vi "Read Joystick.vi"(8 "Joystick Deadbanded Value (default of 0.1)":dbl, 11 "Joystick L 1 DevRef":T1) -> (1 "Joystick L 2 X Axis":dbl, 2 "Joystick L 1 Y Axis":dbl, 3 "Joystick L 1 X Axis":dbl)   [LabVIEW 2014]
uses:
  <vilib>/Rock Robotics/WPI/Joystick/WPI_JoystickDevRef.ctl
  <vilib>/Rock Robotics/WPI/Joystick/WPI_JoystickDeviceEnum.ctl
  Global Variables.vi
  <vilib>/Rock Robotics/WPI/Joystick/WPI_JoystickGetSetRefNum.vi
  <vilib>/Rock Robotics/Network Tables/SD Write Number.vi
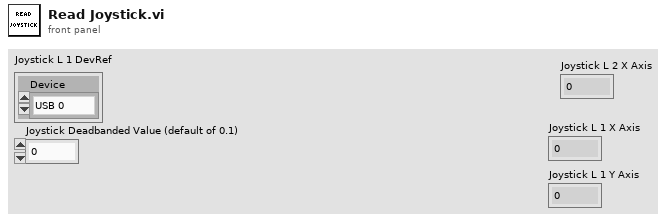
[diagram p1: front panel]
types:
  T1 = typedef "WPI_JoystickDevRef.ctl" = cluster{"Device":T2}
  T2 = typedef "WPI_JoystickDeviceEnum.ctl" = enum16{"USB 0", "USB 1", "USB 2", "USB 3", "USB 4", "USB 5"}
  T3 = cluster{"Buttons[0]":bool, "Buttons[1]":bool, "Buttons[2]":bool, "Buttons[3]":bool, "Buttons[4]":bool, "Buttons[5]":bool, "Buttons[6]":bool, "Buttons[7]":bool, "Buttons[8]":bool}
  T4 = cluster{"Axes[0]":dbl, "Axes[1]":dbl, "Axes[2]":dbl, "Axes[3]":dbl, "Axes[4]":dbl, "Axes[5]":dbl, "Axes[6]":dbl, "Axes[7]":dbl, "Axes[8]":dbl}
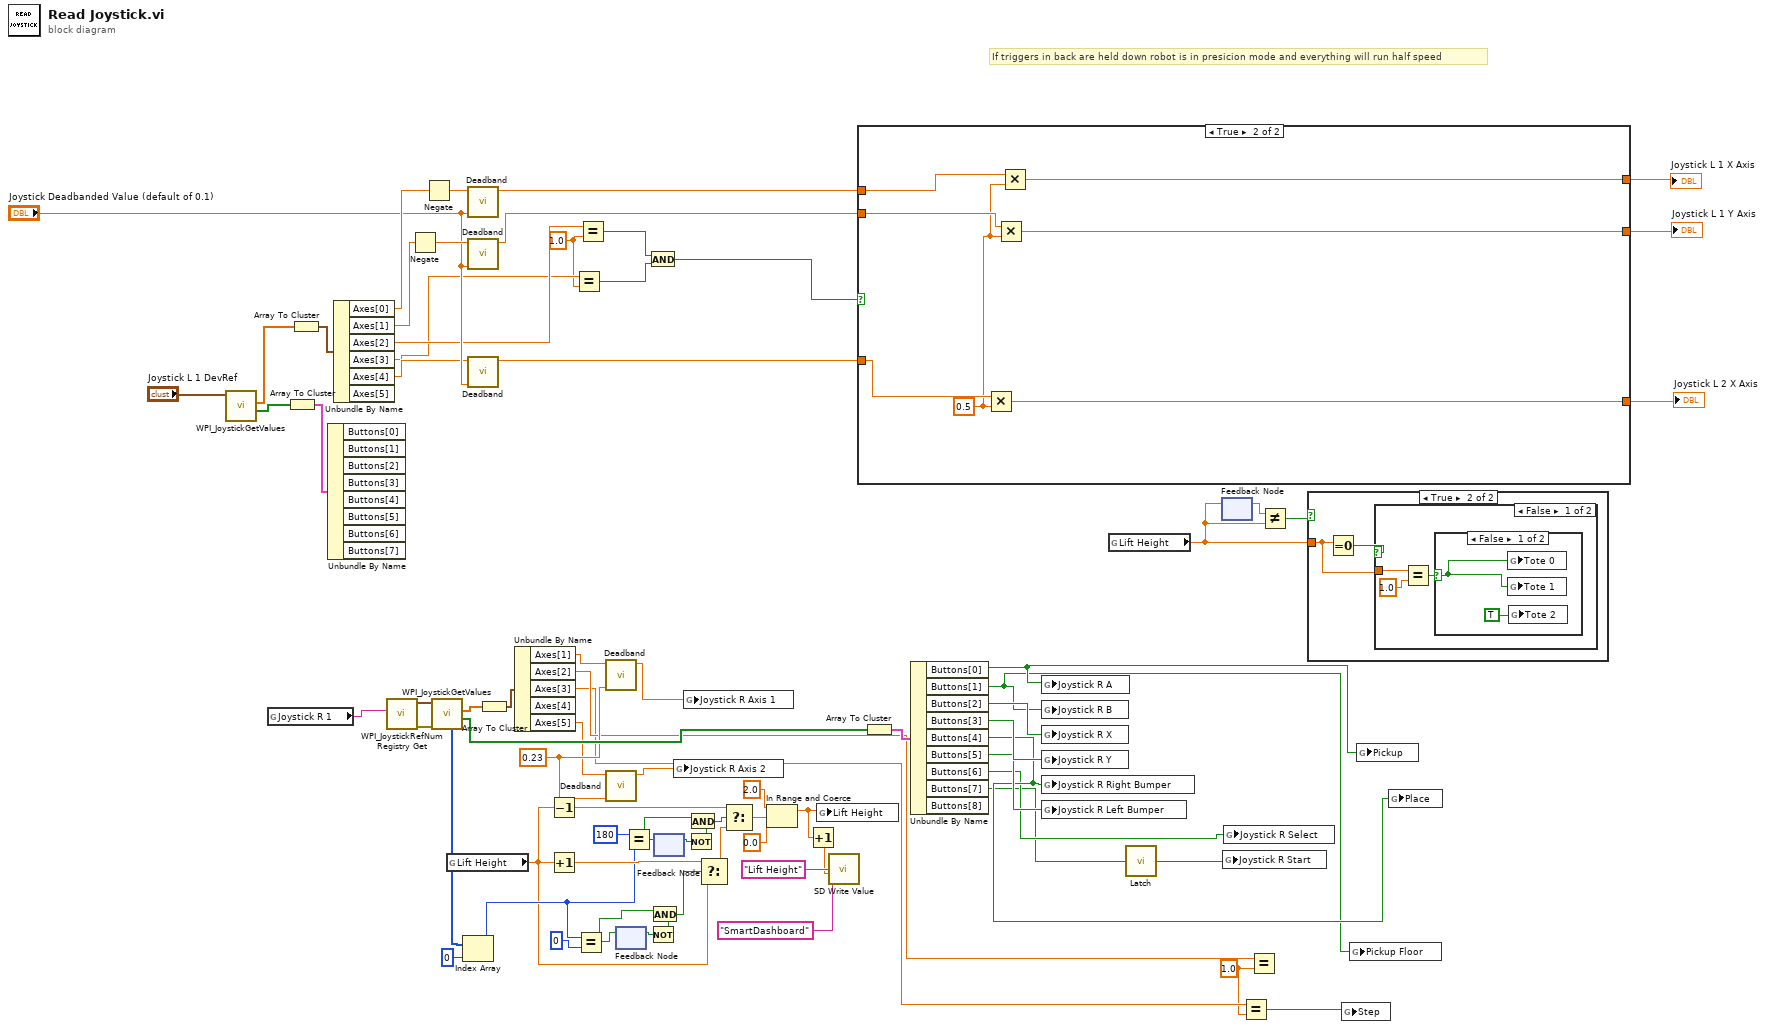
[diagram p0: block diagram]
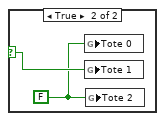
[diagram p3: hidden frame]
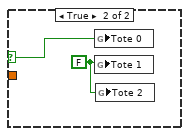
[diagram p4: hidden frame]
diagram:
  w32 = 1.0 ("y")
  w52 = 1.0 ("y")
  w41 = 0.23 ("Value to Deadband (default of 0.1)")
  # "If triggers in back are held down robot is in presicion mode and everything will run half speed"
  n1 = call <vilib>:"WPI_JoystickGetValues.vi"("JoystickDevRef"="Joystick L 1 DevRef") -> ("Buttons"=w72:bool[], "Axes"=w74:dbl[])  [unwired: 6 in, 3 out]
  n2 = global read "Global Variables.vi" "Joystick R 1"() -> (w63:string)
  n3 = Array To Cluster(array=w72) -> (cluster=w71:T3)
  n4 = Array To Cluster(array=w74) -> (cluster=w73:T4)
  n5 = Unbundle By Name(w71) -> ()  [unwired: 8 out]
  n6 = Unbundle By Name(w73) -> ("Axes[0]"=w70:dbl, "Axes[1]"=w67:dbl, "Axes[2]"=w54:dbl, "Axes[3]"=w53:dbl, "Axes[4]"=w55:dbl)  [unwired: 1 out]
  n7 = call <vilib>:"WPI_JoystickRefNum Registry Get.vi"("refnum name"=w63) -> ("error out"=w62:errorcluster, "JoystickDevRef"=w61:T1)  [unwired: 9 in]
  n8 = Negate(x=w67) -> (-x=w68:dbl)
  n9 = Negate(x=w70) -> (-x=w69:dbl)
  n10 = call <vilib>:"WPI_JoystickGetValues.vi"("error in (no error)"=w62, "JoystickDevRef"=w61) -> ("Buttons"=w56:bool[], "Axes"=w64:dbl[], "POVs"=w39:i16[])  [unwired: 5 in, 2 out]
  n11 = global read "Global Variables.vi" "Lift Height"() -> (w6:dbl)
  n12 = Index Array(array=w39, index=0) -> (element=w20:i16)
  n13 = call "Deadband.vi"("Value to Deadband (default of 0.1)"="Joystick Deadbanded Value (default of 0.1)", "Value"=w69) -> ("Deadbanded Value"=w46:dbl)  [unwired: 9 in]
  n14 = call "Deadband.vi"("Value to Deadband (default of 0.1)"="Joystick Deadbanded Value (default of 0.1)", "Value"=w68) -> ("Deadbanded Value"=w47:dbl)  [unwired: 9 in]
  n15 = call "Deadband.vi"("Value to Deadband (default of 0.1)"="Joystick Deadbanded Value (default of 0.1)", "Value"=w55) -> ("Deadbanded Value"=w48:dbl)  [unwired: 9 in]
  n16 = Array To Cluster(array=w64) -> (cluster=w65:T4)
  n17 = Unbundle By Name(w65) -> ("Axes[1]"=w60:dbl, "Axes[2]"=w35:dbl, "Axes[3]"=w33:dbl, "Axes[5]"=w40:dbl)  [unwired: 1 out]
  n18 = Decrement(x=w6) -> (x-1=w21:dbl)
  n19 = Increment(x=w6) -> (x+1=w24:dbl)
  n20 = Equal?(x=w53, y=w52) -> (x = y?=w50:bool)
  n21 = Equal?(x=w20, y=i16 0) -> (x = y?=w10:bool)
  n22 = Equal?(x=w54, y=w52) -> (x = y?=w51:bool)
  n23 = call "Deadband.vi"("Value to Deadband (default of 0.1)"=w41, "Value"=w60) -> ("Deadbanded Value"=w59:dbl)  [unwired: 9 in]
  n24 = call "Deadband.vi"("Value to Deadband (default of 0.1)"=w41, "Value"=w40) -> ("Deadbanded Value"=w42:dbl)  [unwired: 9 in]
  n25 = feedback #1() -> (w11:bool)  [unwired: 1 in]
  n26 = feedback-in #1(w10) -> ()
  n27 = Equal?(x=i16 180 ("y"), y=w20) -> (x = y?=w13:bool)
  n28 = And(x=w51, y=w50) -> (x .and. y?=w49:bool)
  n29 = Not(x=w11) -> (.not. x?=w12:bool)
  n30 = And(x=w10, y=w12) -> (x .and. y?=w9:bool)
  n31 = feedback-in #2(w13) -> ()
  n32 = feedback #2() -> (w15:bool)  [unwired: 1 in]
  n33 = global write "Global Variables.vi" "Joystick R Axis 2"(w42) -> ()
  n34 = global write "Global Variables.vi" "Joystick R Axis 1"(w59) -> ()
  n35 = Not(x=w15) -> (.not. x?=w14:bool)
  n36 = And(x=w13, y=w14) -> (x .and. y?=w16:bool)
  n37 = Select(t=w24, s=w9, f=w6) -> (s? t:f=w25:dbl)
  n38 = Select(t=w21, s=w16, f=w25) -> (s? t:f=w19:dbl)
  n39 = In Range and Coerce(upper limit=2.0, x=w19, lower limit=0.0) -> (coerced(x)=w3:dbl)  [unwired: 1 out]
  n40 = Increment(x=w3) -> (x+1=w2:dbl)
  n41 = global write "Global Variables.vi" "Lift Height"(w3) -> ()
  n42 = call-poly <vilib>:"SD Write Value.vi"("Numeric"=w2, "Table Prefix"="SmartDashboard", "Name"="Lift Height") -> ()  [unwired: 7 in, 2 out]
  n43 = case shown="True" w49 {
    tunnel: w48 -> [w76 w85]
    tunnel: w47 -> [w77 w84]
    tunnel: w46 -> [w78 w82]
    tunnel: [w78 w81] -> w45
    tunnel: [w77 w80] -> w44
    tunnel: [w76 w79] -> w43
    frame False {
    }
    frame True {
      w83 = 0.5 ("y")
      n44 = Multiply(x=w85, y=w83) -> (x*y=w79:dbl)
      n45 = Multiply(x=w84, y=w83) -> (x*y=w80:dbl)
      n46 = Multiply(x=w82, y=w83) -> (x*y=w81:dbl)
    }
  }
  "Joystick L 1 Y Axis" <- w44
  "Joystick L 1 X Axis" <- w45
  "Joystick L 2 X Axis" <- w43
  n47 = Array To Cluster(array=w56) -> (cluster=w57:T3)
  n48 = Unbundle By Name(w57) -> ("Buttons[0]"=w27:bool, "Buttons[1]"=w26:bool, "Buttons[2]"=w58:bool, "Buttons[3]"=w37:bool, "Buttons[4]"=w34:bool, "Buttons[5]"=w36:bool, "Buttons[6]"=w30:bool, "Buttons[7]"=w29:bool)  [unwired: 1 out]
  n49 = global write "Global Variables.vi" "Joystick R A"(w27) -> ()
  n50 = global write "Global Variables.vi" "Joystick R B"(w26) -> ()
  n51 = global write "Global Variables.vi" "Joystick R X"(w58) -> ()
  n52 = global write "Global Variables.vi" "Joystick R Y"(w37) -> ()
  n53 = global write "Global Variables.vi" "Joystick R Right Bumper"(w34) -> ()
  n54 = global write "Global Variables.vi" "Joystick R Left Bumper"(w36) -> ()
  n55 = global read "Global Variables.vi" "Lift Height"() -> (w5:dbl)
  n56 = call "Latch.vi"("Input"=w29) -> ("Output"=w28:bool)
  n57 = feedback-in #3(w5) -> ()
  n58 = feedback #3() -> (w8:dbl)  [unwired: 1 in]
  n59 = global write "Global Variables.vi" "Joystick R Start"(w28) -> ()
  n60 = global write "Global Variables.vi" "Joystick R Select"(w30) -> ()
  n61 = Equal?(x=w33, y=w32) -> (x = y?=w31:bool)
  n62 = Equal?(x=w35, y=w32) -> ()  [unwired: 1 out]
  n63 = Not Equal?(x=w8, y=w5) -> (x != y?=w7:bool)
  n64 = case shown="True" w7 {
    tunnel: w5 -> [_ w86]
    frame False {
    }
    frame True {
      n65 = Equal To 0?(x=w86) -> (x = 0?=w87:bool)
      n66 = case shown="False" w87 {
        selector: w87 -> [_ w96]
        tunnel: w86 -> [w89 _]
        frame False {
          n67 = Equal?(x=w89, y=1.0) -> (x = y?=w90:bool)
          n68 = case shown="False" w90 {
            selector: w90 -> [w91 w94]
            frame False {
              n69 = global write "Global Variables.vi" "Tote 0"(w91) -> ()
              n70 = global write "Global Variables.vi" "Tote 1"(w91) -> ()
              n71 = global write "Global Variables.vi" "Tote 2"(TRUE) -> ()
            }
            frame True {
              w93 = FALSE
              n72 = global write "Global Variables.vi" "Tote 0"(w93) -> ()
              n73 = global write "Global Variables.vi" "Tote 1"(w94) -> ()
              n74 = global write "Global Variables.vi" "Tote 2"(w93) -> ()
            }
          }
        }
        frame True {
          w95 = FALSE
          n75 = global write "Global Variables.vi" "Tote 0"(w96) -> ()
          n76 = global write "Global Variables.vi" "Tote 1"(w95) -> ()
          n77 = global write "Global Variables.vi" "Tote 2"(w95) -> ()
        }
      }
    }
  }
  n78 = global write "Global Variables.vi" "Step"(w31) -> ()
  n79 = global write "Global Variables.vi" "Pickup Floor"(w26) -> ()
  n80 = global write "Global Variables.vi" "Pickup"(w27) -> ()
  n81 = global write "Global Variables.vi" "Place"(w34) -> ()
